vi "Misc Configuration RefOnly.vi"(8 "error in (no error)":errorcluster, 11 "Serial in":refnum<class "Serial.lvclass">) -> (0 "error out":errorcluster, 3 "Serial out":refnum<class "Serial.lvclass">)   [LabVIEW 2021, in "Serial.lvclass"]
uses:
  Serial.lvclass
  <vilib>/Instr/_visa.llb/VISA Configure Serial Port (Instr).vi
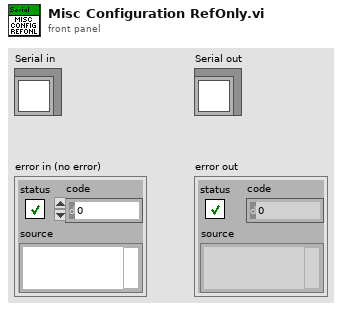
[diagram p1: front panel]
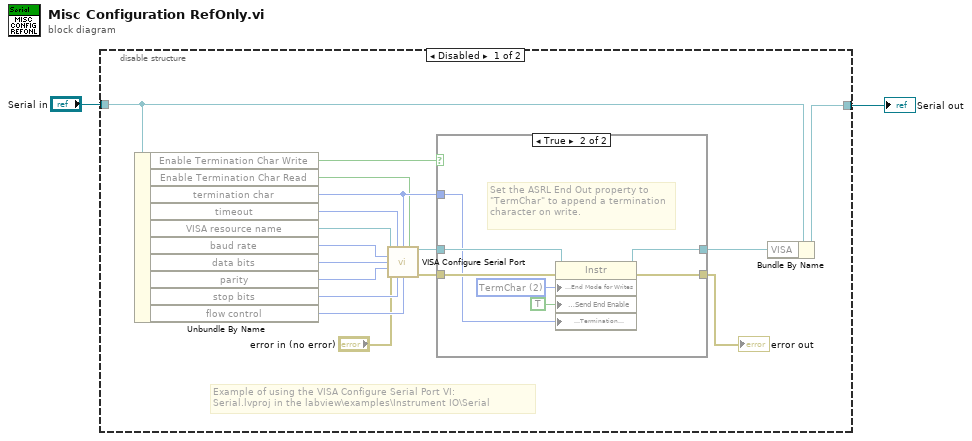
[diagram p0: block diagram]
diagram:
  n1 = disable-structure shown="Disabled" {
    disable-tunnel: [w6 w29] -> w2
    disable-tunnel: "Serial in" -> [w3 w29]
    frame Disabled {
      # "Example of using the VISA Configure Serial Port VI:\nSerial.lvproj in the labview\\examples\\Instrument IO\\Serial"
      n2 = Unbundle By Name(w3) -> ("Enable Termination Char Write"=w16:bool, "Enable Termination Char Read"=w7:bool, "termination char"=w8:u8, "timeout"=w9:u32, "VISA resource name"=w10:refnum<visa-resource-name>, "baud rate"=w11:u32, "data bits"=w12:u16, "parity"=w13:enum16{"None", "Odd", "Even", "Mark", "Space"}, "stop bits"=w14:u16, "flow control"=w15:u16)
      n3 = call-poly "VISA Configure Serial Port"("VISA resource name"=w10, "timeout (10sec)"=w9, "termination char\n(0xA = '\\n' = LF)"=w8, "Enable Termination\nChar (T)"=w7, "baud rate (9600)"=w11, "data bits (8)"=w12, "parity (0:none)"=w13, "error in (no error)"="error in (no error)", "stop bits (10: 1 bit)"=w14, "flow control (0:none)"=w15) -> ("VISA resource name out"=w18:refnum<visa-resource-name>, "error out"=w19:errorcluster)  [unwired: 4 out]
      n4 = case shown="True" w16 {
        tunnel: w19 -> [w20 w28]
        tunnel: w18 -> [w21 w27]
        tunnel: [w20 w24] -> w4
        tunnel: [w21 w23] -> w17
        tunnel: w8 -> [_ w22]
        frame False {
        }
        frame True {
          w26 = u16 2 items=["None", "LastBit", "TermChar", "Break"] ("Serial Settings:Serial End Mode for Writes")
          # "Set the ASRL End Out property to \"TermChar\" to append a termination character on write."
          n5 = property class="Instr"(reference=w27, error in=w28, "Serial Settings:End Mode for Writes"=w26, "Message Based Settings:Send End Enable"=TRUE, "Message Based Settings:Termination Character"=w22) -> (reference out=w23:refnum<visa-resource-name>, error out=w24:errorcluster)
        }
      }
      "error out" <- w4
      n6 = Bundle By Name(cluster=w3, "VISA"=w17) -> (w6:refnum<class "Serial.lvclass">)
    }
    frame Enabled {
    }
  }
  "Serial out" <- w2
